vi "SETUP TEST CONDITIONS(SubVI) RT.vi"(6 "setup time":u16, 7 "capacity usable(Ah)":dbl, 8 "setup value":dbl, 9 "setup test by":u16) -> (0 "Current(A)":dbl, 1 "Time(s)":dbl, 2 "C discharge":bool, 3 "Current":bool, 4 "C discharge":dbl, 5 "Time":bool)   [LabVIEW 2017]
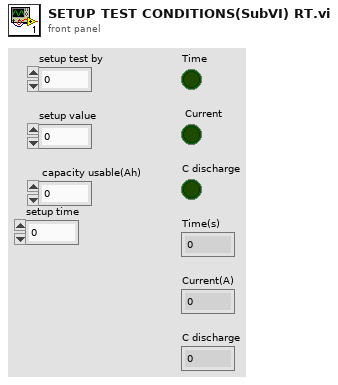
[diagram p1: front panel]
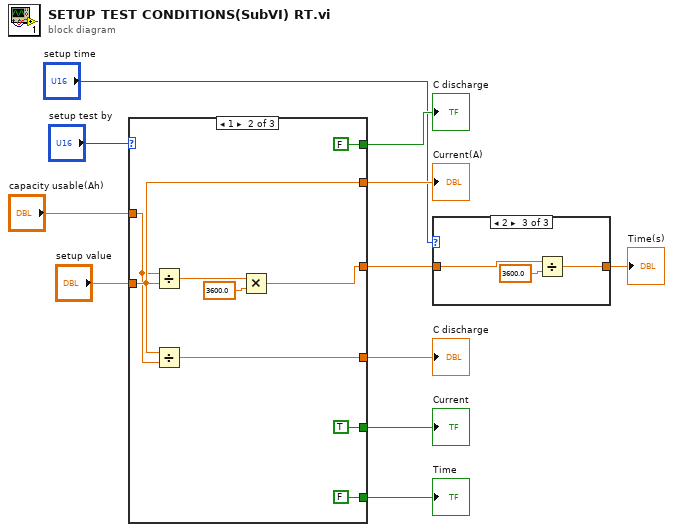
[diagram p0: block diagram]
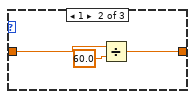
[diagram p3: hidden frame]
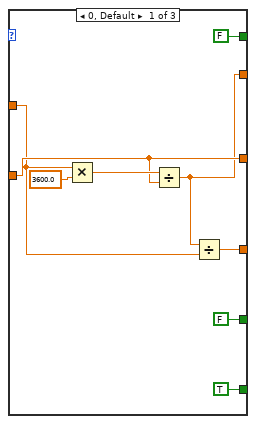
[diagram p4: hidden frame]
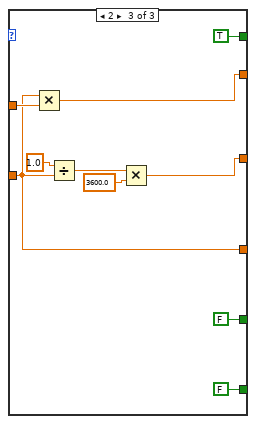
[diagram p5: hidden frame]
diagram:
  n1 = case shown="1" "setup test by" {
    tunnel: "capacity usable(Ah)" -> [w13 w21 w36]
    tunnel: "setup value" -> [w15 w22 w33]
    tunnel: [TRUE FALSE FALSE] -> w7
    tunnel: [FALSE TRUE FALSE] -> w8
    tunnel: [FALSE FALSE TRUE] -> w9
    tunnel: [w15 w24 w30] -> w1
    tunnel: [w12 w22 w35] -> w10
    tunnel: [w14 w23 w33] -> w11
    frame 0, Default {
      n2 = Multiply(x=w13, y=3600.0) -> (x*y=w16:dbl)
      n3 = Divide(x=w16, y=w15) -> (x/y=w12:dbl)
      n4 = Divide(x=w12, y=w13) -> (x/y=w14:dbl)
    }
    frame 1 {
      n5 = Divide(x=w21, y=w22) -> (x/y=w26:dbl)
      n6 = Divide(x=w22, y=w21) -> (x/y=w23:dbl)
      n7 = Multiply(x=w26, y=3600.0) -> (x*y=w24:dbl)
    }
    frame 2 {
      n8 = Multiply(x=w33, y=w36) -> (x*y=w35:dbl)
      n9 = Divide(x=1.0, y=w33) -> (x/y=w32:dbl)
      n10 = Multiply(x=w32, y=3600.0) -> (x*y=w30:dbl)
    }
  }
  "Time" <- w7
  "Current" <- w8
  "C discharge" <- w9
  "Current(A)" <- w10
  "C discharge" <- w11
  n11 = case shown="2" "setup time" {
    tunnel: [w40 w42 w45] -> w2
    tunnel: w1 -> [w40 w43 w46]
    frame 0, Default {
    }
    frame 1 {
      n12 = Divide(x=w43, y=60.0) -> (x/y=w42:dbl)
    }
    frame 2 {
      n13 = Divide(x=w46, y=3600.0) -> (x/y=w45:dbl)
    }
  }
  "Time(s)" <- w2
